vi "Show Splash Screen.vi"(8 "error in":errorcluster, 11 "Base Software in":refnum<class "Base Software.lvclass">) -> (0 "error out":errorcluster, 3 "Base Software out":refnum<class "Base Software.lvclass">)   [LabVIEW 2019, in "Base Software.lvlib" / "Main.lvlib" / "Base Software.lvclass"]
uses:
  Project/Base Software.lvclass
  C:/Users/Public/Documents/Development/builds/Engine/Engine.lvlibp/Project/Engine.lvclass
  Project/Base Software.lvclass/Base Software.ctl
  Accessors/StateMachine/Read State.vi
  Accessors/GUI/Read Prime Panel ref.vi
  builds/Engine/Engine.lvlibp/Accessors/Read Directory.vi
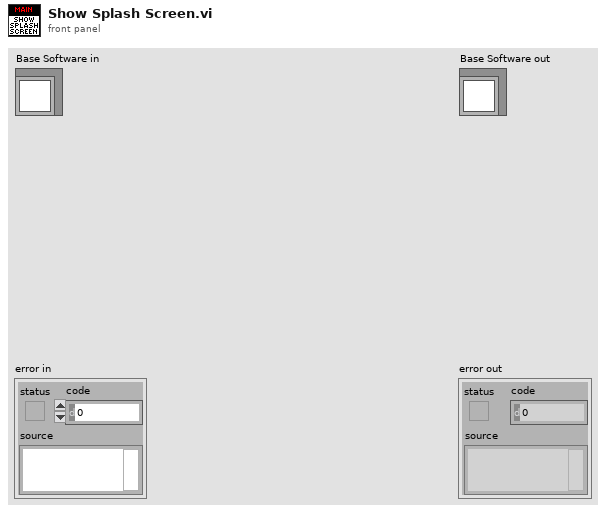
[diagram p1: front panel]
types:
  T1 = typedef "Engine.lvlibp/Engine.lvclass/System Status.ctl" = enum16{"Logged Off", "UUT_Info_Missing", "Idle", "Error", "Warning", "Loading", "Config", "Manual", "Automation", "Report_View", "Previous"}
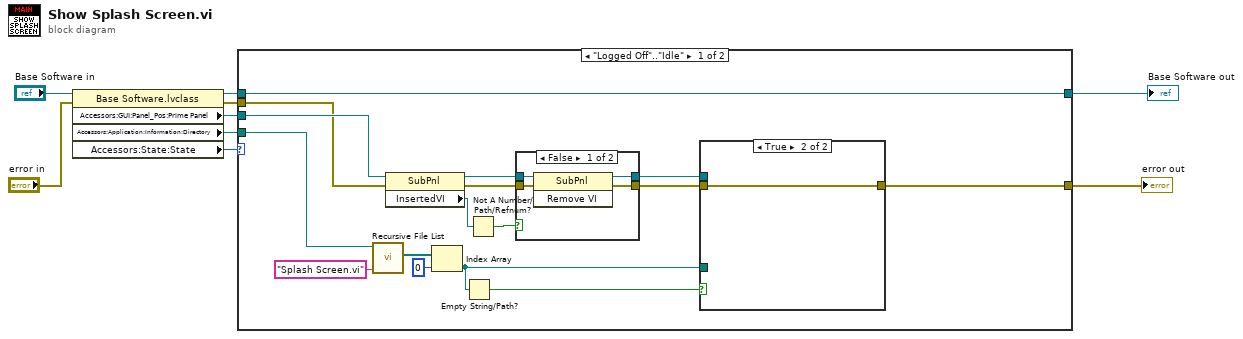
[diagram p0: block diagram]
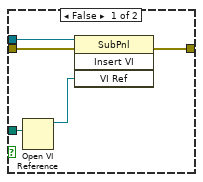
[diagram p2: hidden frame]
diagram:
  n1 = property class="Base Software.lvclass"(reference="Base Software in", error in="error in") -> (reference out=w2:refnum<class "Base Software.lvclass">, error out=w5:errorcluster, "Accessors:GUI:Panel_Pos:Prime Panel"=w8:refnum<vi>, "Accessors:Application:Information:Directory"=w7:path, "Accessors:State:State"=w3:T1)
  n2 = case shown="\"Logged Off\"..\"Idle\"" w3 {
    tunnel: w8 -> [w21 _]
    tunnel: w7 -> [w12 _]
    tunnel: w5 -> [w20 w38]
    tunnel: [w17 w38] -> w4
    tunnel: w2 -> [w16 w39]
    tunnel: [w16 w39] -> w1
    frame "Logged Off".."Idle" {
      n3 = call <vilib>:"Recursive File List.vi"("pattern"="Splash Screen.vi" ("name or relative path"), "Folder Path"=w12) -> ("All Files in Dir"=w14:path[])  [unwired: 5 in, 4 out]
      n4 = property class="SubPnl"(reference=w21, error in=w20) -> (reference out=w24:refnum<vi>, error out=w19:errorcluster, "InsertedVI"=w22:refnum<vi>)
      n5 = Index Array(array=w14, index=0) -> (element=w11:path)
      n6 = Empty String/Path?(string/path=w11) -> (empty?=w10:bool)
      n7 = Not A Number/Path/Refnum?(number/path/refnum=w22) -> (NaN/Path/Refnum?=w23:bool)
      n8 = case shown="False" w23 {
        tunnel: w24 -> [w35 w37]
        tunnel: [w34 w37] -> w25
        tunnel: w19 -> [w33 w36]
        tunnel: [w32 w36] -> w18
        frame False {
          n9 = invoke class="SubPnl" method="Remove VI"(reference=w35, error in=w33) -> (reference out=w34:refnum<vi>, error out=w32:errorcluster)  [unwired: 1 in, 1 out]
        }
        frame True {
        }
      }
      n10 = case shown="True" w10 {
        tunnel: w25 -> [w30 _]
        tunnel: w18 -> [w28 w31]
        tunnel: [w27 w31] -> w17
        tunnel: w11 -> [w26 _]
        frame False {
          n11 = Open VI Reference(vi path=w26) -> (vi reference=w29:refnum<vi>)  [unwired: 5 in, 1 out]
          n12 = invoke class="SubPnl" method="Insert VI"(reference=w30, error in=w28, "VI Ref"=w29) -> (error out=w27:errorcluster)  [unwired: 1 in, 3 out]
        }
        frame True {
        }
      }
    }
    frame Default {
    }
  }
  "error out" <- w4
  "Base Software out" <- w1
